vi "NF LI56xx u_crackToStr.vi"(0 "input string":string) -> (14 "output string":string)   [LabVIEW 2019]
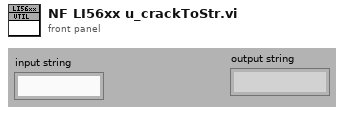
[diagram p1: front panel]
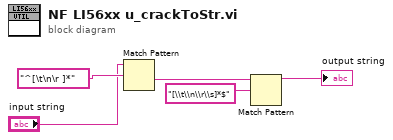
[diagram p0: block diagram]
diagram:
  n1 = Match Pattern(string="input string", regular expression="^[\t\n\r ]*" ("正規表現")) -> (after substring=w3:string)  [unwired: 1 in, 3 out]
  n2 = Match Pattern(string=w3, regular expression="[\\t\\n\\r\\s]*$" ("正規表現")) -> (before substring=→"output string":string)  [unwired: 1 in, 3 out]
